vi "(SubVI) Get Time from FEC file.vi"(6 "Folder path":path, 7 "path":path) -> (0 "sec":i32, 1 "min":i32, 2 "hr":i32, 3 "hr/min/s":i32)   [LabVIEW 2014]
panel:
  out "substring":string
  out "before substring":string
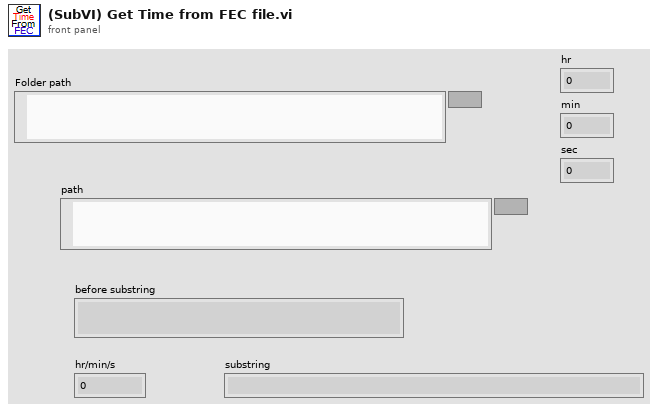
[diagram p1: front panel]
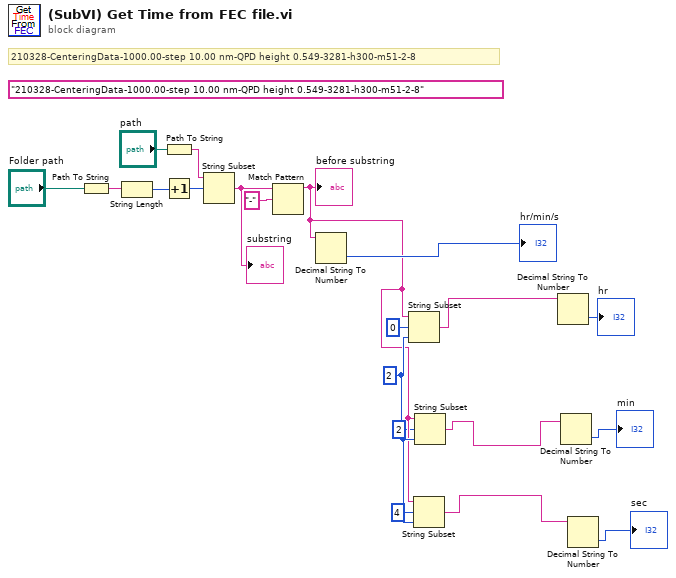
[diagram p0: block diagram]
diagram:
  w11 = 2 ("length (rest)")
  (unwired) "210328-CenteringData-1000.00-step 10.00 nm-QPD height 0.549-3281-h300-m51-2-8" ("match substring")
  # "210328-CenteringData-1000.00-step 10.00 nm-QPD height 0.549-3281-h300-m51-2-8"
  n1 = Path To String(path="Folder path") -> (string=w16:string)
  n2 = String Length(string=w16) -> (length=w14:i32)
  n3 = Path To String(path="path") -> (string=w15:string)
  n4 = Increment(x=w14) -> (x+1=w13:i32)
  n5 = String Subset(string=w15, offset (0)=w13) -> (substring=w7:string)  [unwired: 1 in]
  "substring" <- w7
  n6 = Match Pattern(string=w7, regular expression="-" ("match substring")) -> (before substring=w10:string)  [unwired: 1 in, 3 out]
  "before substring" <- w10
  n7 = Decimal String To Number(string=w10) -> (number=→"hr/min/s":i32)  [unwired: 2 in, 1 out]
  n8 = String Subset(string=w10, offset (0)=0, length (rest)=w11) -> (substring=w6:string)
  n9 = String Subset(string=w10, offset (0)=4, length (rest)=w11) -> (substring=w4:string)
  n10 = String Subset(string=w10, offset (0)=2, length (rest)=w11) -> (substring=w5:string)
  n11 = Decimal String To Number(string=w6) -> (number=→"hr":i32)  [unwired: 2 in, 1 out]
  n12 = Decimal String To Number(string=w5) -> (number=→"min":i32)  [unwired: 2 in, 1 out]
  n13 = Decimal String To Number(string=w4) -> (number=→"sec":i32)  [unwired: 2 in, 1 out]
